vi "Autosetup.vi"(8 "error in (no error)":errorcluster, 11 "VISA resource name":refnum<visa-resource-name>) -> (0 "error out":errorcluster, 3 "VISA resource name out":refnum<visa-resource-name>)   [LabVIEW 2009, in "Agilent 8000 Series.lvlib"]
doc: "Causes the oscilloscope to evaluate all input waveforms and find the optimum conditions for displaying the waveform."
uses:
  Agilent 8000 Series.lvlib
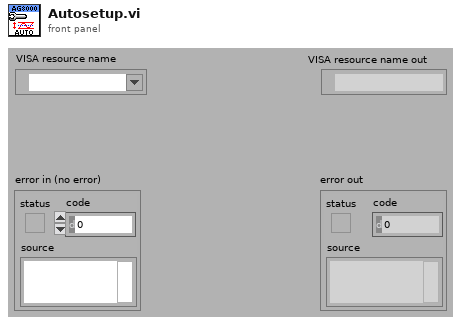
[diagram p1: front panel]
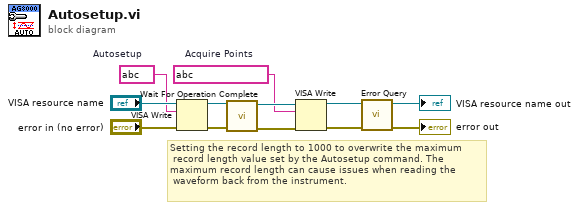
[diagram p0: block diagram]
diagram:
  w1 = string ?  # Acquire Points
  w10 = string ?  # Autosetup
  # "Setting the record length to 1000 to overwrite the maximum\n record length value set by the Autosetup command. The \nmaximum record length can cause issues when reading the\n waveform back from the instrument."
  n1 = VISA Write(VISA resource name="VISA resource name", write buffer=w10, error in (no error)="error in (no error)") -> (VISA resource name out=w7:refnum<visa-resource-name>, error out=w6:errorcluster)  [unwired: 1 out]
  n2 = call "Wait For Operation Complete.vi"("error in (no error)"=w6, "VISA resource name"=w7) -> ("error out"=w4:errorcluster, "VISA resource name out"=w5:refnum<visa-resource-name>)  [unwired: 8 in]
  n3 = VISA Write(VISA resource name=w5, write buffer=w1, error in (no error)=w4) -> (VISA resource name out=w2:refnum<visa-resource-name>, error out=w3:errorcluster)  [unwired: 1 out]
  n4 = call "Error Query.vi"("error in (no error)"=w3, "VISA resource name"=w2) -> ("error out"=→"error out":errorcluster, "VISA resource name out"=→"VISA resource name out":refnum<visa-resource-name>)  [unwired: 6 in, 2 out]
